vi "firstKickAdjustPosition.vi"(6 "Dist":dbl, 8 "error in (no error)":errorcluster, 9 "Orientation":dbl, 10 "Dest":dbl[](array[numeric]), 11 "WaitBallTrajSkill in":refnum<class "WaitBallTrajSkill.lvclass">) -> (0 "error out":errorcluster, 2 "AdjustDest":dbl[](array[numeric]), 3 "WaitBallTrajSkill out":refnum<class "WaitBallTrajSkill.lvclass">)   [LabVIEW 2024, in "WaitBallTrajSkill.lvclass"]
uses:
  WaitBallTrajSkill.lvclass
  <vilib>/Analysis/coordinate.llb/2D Cartesian Coordinate Rotation (Scalar).vi
  <vilib>/Analysis/NI_AALPro.lvlib
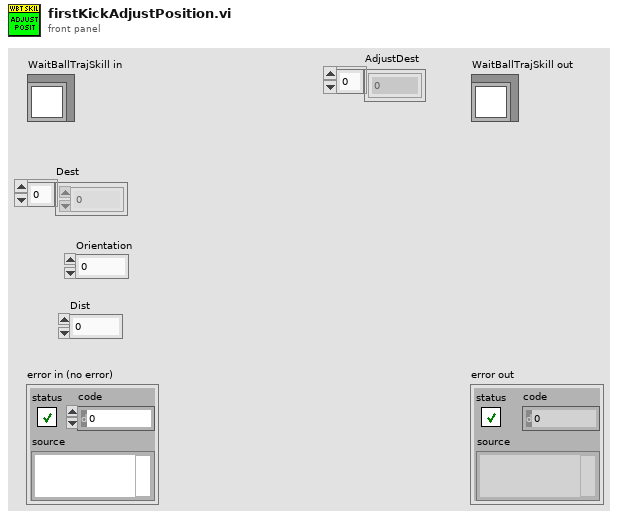
[diagram p1: front panel]
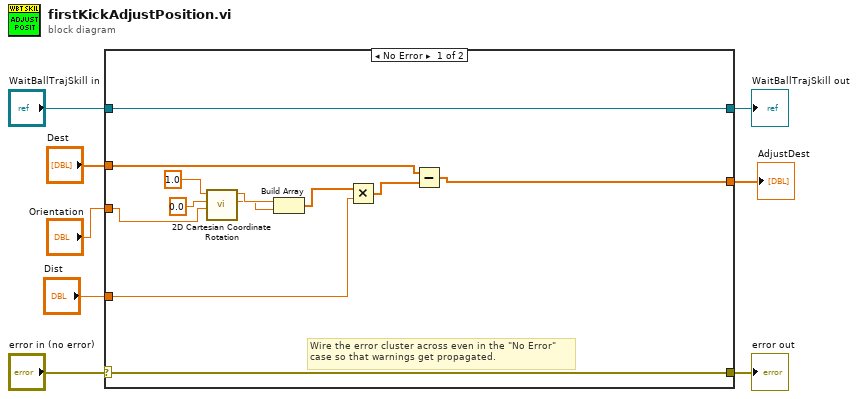
[diagram p0: block diagram]
diagram:
  n1 = case shown="No Error" "error in (no error)" {
    selector: "error in (no error)" -> [w19 w22]
    tunnel: [w19 w22] -> w7
    tunnel: [w20 w21] -> w5
    tunnel: "WaitBallTrajSkill in" -> [w20 w21]
    tunnel: "Orientation" -> [w16 _]
    tunnel: "Dist" -> [w12 _]
    tunnel: "Dest" -> [w10 _]
    tunnel: [w9 _] -> w1
    frame No Error {
      # "Wire the error cluster across even in the \"No Error\"\ncase so that warnings get propagated."
      n2 = call-poly <vilib>:"2D Cartesian Coordinate Rotation.vi"("theta"=w16, "y"=0.0, "x"=1.0) -> ("y out"=w14:dbl, "x out"=w15:dbl)  [unwired: 6 in, 1 out]
      n3 = Build Array(w15, w14) -> (w13:dbl[])
      n4 = Multiply(x=w13, y=w12) -> (x*y=w11:dbl[])
      n5 = Subtract(x=w10, y=w11) -> (x-y=w9:dbl[])
    }
    frame Error {
    }
  }
  "error out" <- w7
  "WaitBallTrajSkill out" <- w5
  "AdjustDest" <- w1
